vi "DMM DCCM Configure and Measure Only in a Loop.vi"() -> ()   [LabVIEW 2021]
uses:
  DMM_DC-RMS Current Measurement/Typedefs/Function Settings.ctl
  <instrlib>/niDMM/nidmm.llb/niDMM Resolution in Digits.ctl
  DMM_DC-RMS Current Measurement/Typedefs/Timing & Trigger Settings.ctl
  <instrlib>/niDMM/nidmm.llb/niDMM Trigger.ctl
  <instrlib>/niDMM/nidmm.llb/niDMM Slope.ctl
  DMM_DC-RMS Current Measurement/Typedefs/Measurement.ctl
  DMM_DC-RMS Current Measurement/Typedefs/DMM Execution Settings.ctl
  <instrlib>/niDMM/nidmm.llb/niDMM Powerline Frequency.ctl
  Common/Typedefs/Execution Options - Measure.ctl
  DMM_DC-RMS Current Measurement/DMM_DC-RMS Current Measurement.lvlib
panel:
  out "error out":errorcluster
  out "DMM Execution Settings":T1={"Absolute\nResolution"=0.0, "Input Resistance\n(Ohm)"=0.0, "Digits\nResolution"=0.0, "Range"=0.0, "Minimum\nFrequency (Hz)"=0.0, "Aperture\nTime (s)"=0.0, "Auto Range\nValue"=0.0, "Settle\nTime (s)"=0.0, "Function"=3} {"Function" items=["DC Volts"=1, "AC Volts"=2, "DC Current"=3, "AC Current"=4, "2-Wire Resistance"=5, "4-Wire Resistance"=101, "Frequency"=104, "Period"=105, "AC Volts DC Coupled"=1001, "Diode"=1002, "Waveform Voltage"=1003, "Waveform Current"=1004, "Capacitance"=1005, "Inductance"=1006, "Temperature"=108]; "Absolute\nResolution" format="%#_6p"; "Input Resistance\n(Ohm)" format="%#_6p"; "Range" format="%#_6p"; "Minimum\nFrequency (Hz)" format="%#_6p"; "Aperture\nTime (s)" format="%#_6p"; "Auto Range\nValue" format="%#_6p"; "Settle\nTime (s)" format="%#_6p"}
  out "Measurement":T2={"Measured Value"=0.0, "Out of Range"=FALSE, "Unit"="A(dc)", "Measurement"="0.0000mA (dc)"} {"Measured Value" format="%^#_9e"}
  in  "Timing & Trigger Settings":T3={"AC Min Frequency (Hz)"=40.0, "Aperture Time (s)"=-1.0, "Settle Time (s)"=-1.0, "Trigger Settings"={"Trigger Delay (sec)"=-1.0, "Enable Trigger?"=FALSE, "Trigger Source"=enum."Immediate", "Slope"=enum."Rising Edge"}} caption="Timing and Trigger Settings" {"Trigger Settings"."Trigger Delay (sec)" format="%.4f"; "AC Min Frequency (Hz)" format="%.2f"}
  in  "Function Settings":T6={"Range and Function"=enum."DC Current Auto Range", "Resolution in Digits"=5.5} {"Resolution in Digits" items=["3 1/2"=3.5, "4 1/2"=4.5, "5 1/2"=5.5, "6 1/2"=6.5, "7 1/2"=7.5]}
  in  "DMM Resource Name":refnum<k15>
  in  "Stop Button":bool
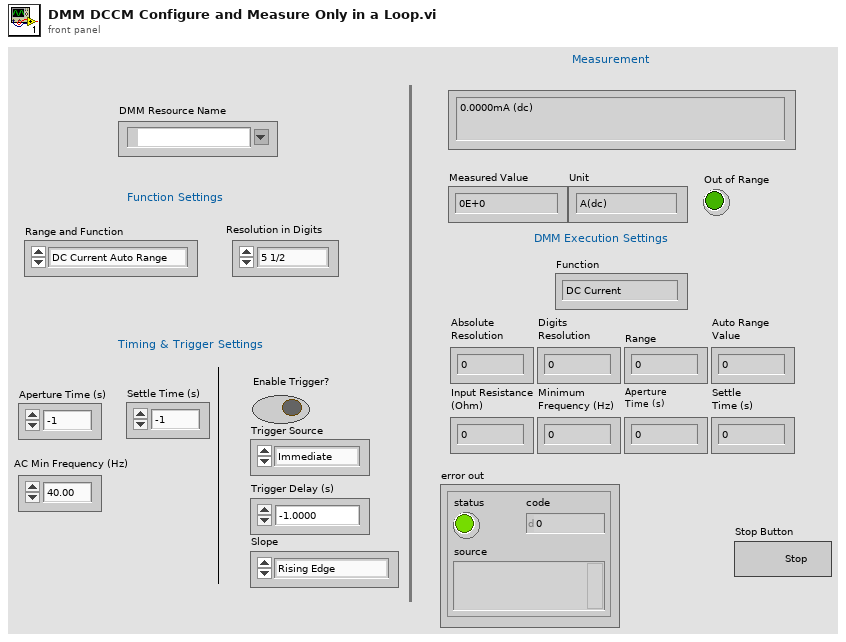
[diagram p1: front panel]
types:
  T1 = typedef "DMM_DC-RMS Current Measurement.lvlib/DMM Execution Settings.ctl" = cluster{"Absolute\nResolution":dbl, "Input Resistance\n(Ohm)":dbl, "Digits\nResolution":dbl, "Range":dbl, "Minimum\nFrequency (Hz)":dbl, "Aperture\nTime (s)":dbl, "Auto Range\nValue":dbl, "Settle\nTime (s)":dbl, "Function":i32}
  T2 = typedef "DMM_DC-RMS Current Measurement.lvlib/Measurement.ctl" = cluster{"Measured Value":dbl, "Out of Range":bool, "Unit":string, "Measurement":string}
  T3 = typedef "DMM_DC-RMS Current Measurement.lvlib/Timing & Trigger Settings.ctl" = cluster{"AC Min Frequency (Hz)":dbl, "Aperture Time (s)":dbl, "Settle Time (s)":dbl, "Trigger Settings":cluster{"Trigger Delay (sec)":dbl, "Enable Trigger?":bool, "Trigger Source":T4, "Slope":T5}}
  T4 = typedef "niDMM Trigger.ctl" = enum16{"Immediate", "External", "TTL 0", "TTL 1", "TTL 2", "TTL 3", "TTL 4", "TTL 5", "TTL 6", "Software", "TTL 7", "PXI Star", "LBR Trig 1", "Aux Trig 1"}
  T5 = typedef "niDMM Slope.ctl" = enum16{"Rising Edge", "Falling Edge"}
  T6 = typedef "DMM_DC-RMS Current Measurement.lvlib/Function Settings.ctl" = cluster{"Range and Function":enum16{"DC Current Auto Range", "DC 1 uA", "DC 10 uA", "DC 100 uA", "DC 1 mA", "DC 10 mA", "DC 20 mA", "DC 100 mA", "DC 200 mA", "DC 1 A", "DC 3 A", "   ", "AC Current Auto Range", "AC 100 uA", "AC 1 mA", "AC 10 mA", "AC 100 mA", "AC 500 mA", "AC 1 A", "AC 3 A"}, "Resolution in Digits":T7}
  T7 = typedef "niDMM Resolution in Digits.ctl" = dbl
  T8 = typedef "Execution Options - Measure.ctl" = enum16{"Configure & Measure", "Configure only", "Measure only"}
  T9 = typedef "niDMM Powerline Frequency.ctl" = enum16{"60 Hz", "50 Hz"}
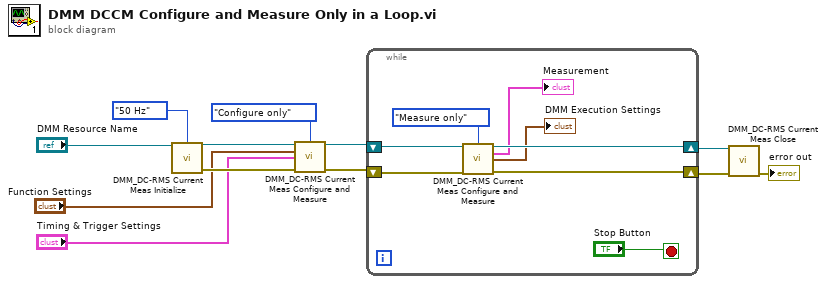
[diagram p0: block diagram]
diagram:
  n1 = call "DMM_DC-RMS Current Meas Initialize.vi"("DMM Resource Name"="DMM Resource Name", "Powerline Frequency"=niDMM_Powerline_Frequency."50 Hz") -> ("DMM Handle Out"=w10:refnum<k15>, "error out"=w9:errorcluster)  [unwired: 12 in]
  n2 = call "DMM_DC-RMS Current Meas Configure and Measure.vi"("DMM Handle In"=w10, "Execution Option"=Execution_Options_-_Measure."Configure only", "Function Settings"="Function Settings", "Timing & Trigger Settings"="Timing & Trigger Settings", "error in"=w9) -> ("DMM Handle Out"=w8:refnum<k15>, "error out"=w7:errorcluster)  [unwired: 7 in, 2 out]
  n3 = while {
    shift-right: [w16] -> w3
    shift-left: w8 -> [w19]
    shift-right: [w15] -> w2
    shift-left: w7 -> [w18]
    stop <- "Stop Button" stop-if-true
    n4 = call "DMM_DC-RMS Current Meas Configure and Measure.vi"("DMM Handle In"=w19, "Execution Option"=Execution_Options_-_Measure."Measure only", "error in"=w18) -> ("DMM Handle Out"=w16:refnum<k15>, "Measurement"=→"Measurement":T2, "DMM Execution Settings"=→"DMM Execution Settings":T1, "error out"=w15:errorcluster)  [unwired: 9 in]
  }
  n5 = call "DMM_DC-RMS Current Meas Close.vi"("DMM Handle In"=w3, "error in"=w2) -> ("error out"=→"error out":errorcluster)  [unwired: 13 in]
